vi "Scan Setup.vi"(8 "error in (no error)":errorcluster, 11 "Temperature Control in":refnum<class "Temperature Control.lvclass">) -> (0 "error out":errorcluster, 3 "Temperature Control out":refnum<class "Temperature Control.lvclass">)   [LabVIEW 2009, in "Temperature Control.lvclass"]
doc: "(Dynamic) Send commands to configure the instrument based on the class member fields."
uses:
  Temperature Control.lvclass
  Reader/Reader.lvclass
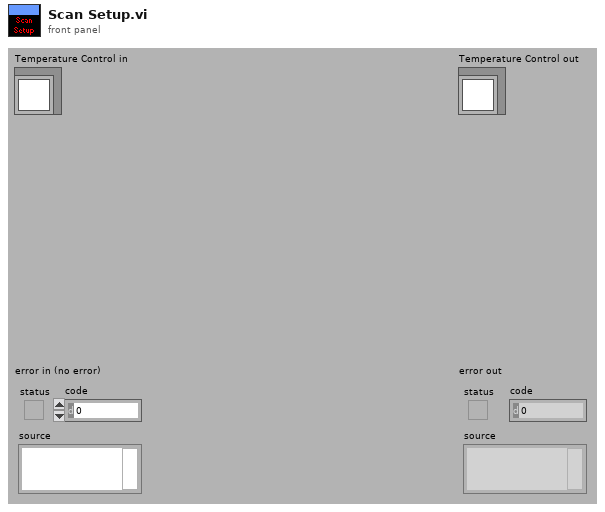
[diagram p1: front panel]
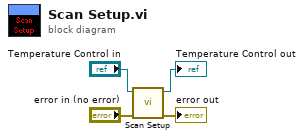
[diagram p0: block diagram]
diagram:
  n1 = call-parent "Scan Setup.vi"("error in (no error)"="error in (no error)", "Reader in"="Temperature Control in") -> ("error out"=→"error out":errorcluster, "Reader out"=→"Temperature Control out":refnum<class "Temperature Control.lvclass">)  [unwired: 8 in]
